vi "Configure Trigger Polarity.vi"(7 "Trigger Polarity Positive (T)":bool=TRUE, 8 "error in (no error)":errorcluster, 11 "VISA resource name":refnum<visa-resource-name>) -> (0 "error out":errorcluster, 3 "VISA resource name out":refnum<visa-resource-name>)   [LabVIEW 2020, in "QuPMXdriver.lvlib"]
doc: "Configures trigger polarity to postive or negative."
uses:
  QuPMXdriver.lvlib
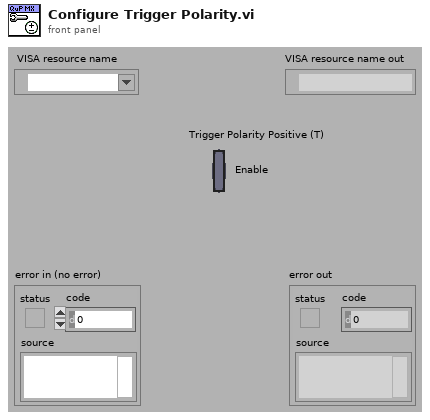
[diagram p1: front panel]
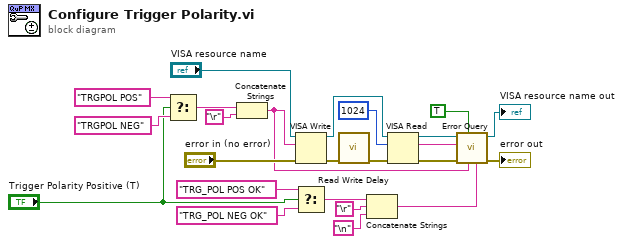
[diagram p0: block diagram]
diagram:
  n1 = Select(t="TRGPOL POS" ("write buffer"), s="Trigger Polarity Positive (T)", f="TRGPOL NEG" ("write buffer")) -> (s? t:f=w18:string)
  n2 = Concatenate Strings(w18, "\r") -> (w10:string)
  n3 = VISA Write(VISA resource name="VISA resource name", write buffer=w10, error in (no error)="error in (no error)") -> (VISA resource name out=w13:refnum<visa-resource-name>, error out=w15:errorcluster)  [unwired: 1 out]
  n4 = Select(t="TRG_POL POS OK" ("write buffer"), s="Trigger Polarity Positive (T)", f="TRG_POL NEG OK" ("write buffer")) -> (s? t:f=w6:string)
  n5 = call "Read Write Delay.vi"("error in"=w15) -> ("error out"=w14:errorcluster)  [unwired: 10 in]
  n6 = Concatenate Strings(w6, "\r", "\n") -> (w1:string)
  n7 = VISA Read(VISA resource name=w13, byte count=u32 1024, error in (no error)=w14) -> (VISA resource name out=w12:refnum<visa-resource-name>, read buffer=w9:string, error out=w8:errorcluster)  [unwired: 1 out]
  n8 = call "Error Query.vi"("Expected read buffer"=w1, "Last command"=w10, "Ignore empty sequence? (T)"=TRUE, "error in (no error)"=w8, "Read buffer"=w9, "VISA resource name"=w12) -> ("error out"=→"error out":errorcluster, "VISA resource name out"=→"VISA resource name out":refnum<visa-resource-name>)  [unwired: 4 in]
